vi "Strtok, Four Doubles.vi"(0 "delimiters (\\s\\t\\r\\n=)":string=" \t\r\n=", 1 "offset":i32, 2 "input string":string="2.3 745") -> (3 "x4":dbl=nan format="%.2f", 4 "x3":dbl=nan format="%.2f", 5 "x 2":dbl=nan format="%.2f", 6 "x1":dbl=nan format="%.2f")   [LabVIEW 2020]
doc: "Scans the input string, starting at offset, for tokens, and outputs four double precision floating point values."
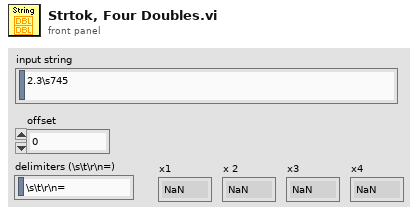
[diagram p1: front panel]
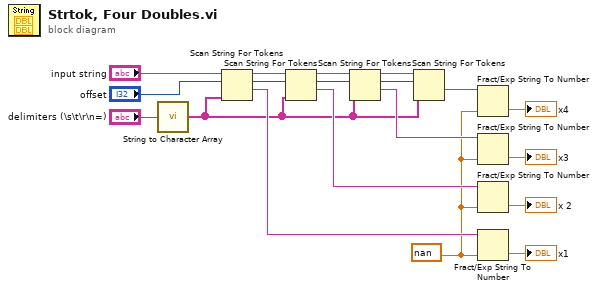
[diagram p0: block diagram]
diagram:
  w8 = nan
  n1 = call "String to Character Array.vi"("input string"="delimiters (\\s\\t\\r\\n=)") -> ("character array"=w3:string[])
  n2 = Scan String For Tokens(6:w3, 8:"offset", 9:"input string") -> (1:w16:string, 2:w17:i32, 3:w18:string)  [unwired: 3 in, 1 out]
  n3 = Scan String For Tokens(6:w3, 8:w17, 9:w18) -> (1:w9:string, 2:w13:i32, 3:w15:string)  [unwired: 3 in, 1 out]
  n4 = Scan String For Tokens(6:w3, 8:w13, 9:w15) -> (1:w10:string, 2:w12:i32, 3:w14:string)  [unwired: 3 in, 1 out]
  n5 = Scan String For Tokens(6:w3, 8:w12, 9:w14) -> (1:w11:string)  [unwired: 3 in, 3 out]
  n6 = Fract/Exp String To Number(string=w11, default (0 dbl)=w8) -> (number=→"x4":dbl)  [unwired: 2 in, 1 out]
  n7 = Fract/Exp String To Number(string=w10, default (0 dbl)=w8) -> (number=→"x3":dbl)  [unwired: 2 in, 1 out]
  n8 = Fract/Exp String To Number(string=w9, default (0 dbl)=w8) -> (number=→"x 2":dbl)  [unwired: 2 in, 1 out]
  n9 = Fract/Exp String To Number(string=w16, default (0 dbl)=w8) -> (number=→"x1":dbl)  [unwired: 2 in, 1 out]
